vi "Updater Install DIAdem 2011.vi"(8 "error in (no error)":errorcluster, 11 "Spartan Install Path":path) -> (0 "error out":errorcluster)   [LabVIEW 2011]
uses:
  <vilib>/registry/registry.llb/Read Registry Value Simple STR.vi
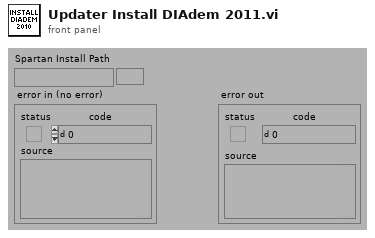
[diagram p1: front panel]
types:
  T1 = typedef "Registry refnum.ctl" = refnum<k1>
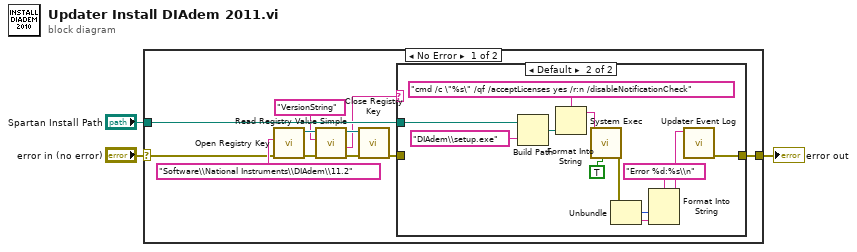
[diagram p0: block diagram]
diagram:
  n1 = case shown="No Error" "error in (no error)" {
    selector: "error in (no error)" -> [w4 w28]
    tunnel: [w14 w28] -> w3
    tunnel: "Spartan Install Path" -> [w13 _]
    frame No Error {
      n2 = call <vilib>:"Open Registry Key.vi"("error in (no error)"=w4, "subkey"="Software\\National Instruments\\DIAdem\\11.2") -> ("error out"=w10:errorcluster, "refnum out"=w9:T1)  [unwired: 8 in]
      n3 = call-poly <vilib>:"Read Registry Value Simple.vi"("error in (no error)"=w10, "value"="VersionString", "refnum"=w9) -> ("error out"=w6:errorcluster, "String/Binary data"=w5:string, "refnum out"=w7:T1)  [unwired: 3 in, 1 out]
      n4 = call <vilib>:"Close Registry Key.vi"("error in (no error)"=w6, "refnum"=w7) -> ("error out"=w12:errorcluster)  [unwired: 5 in]
      n5 = case shown="Default" w5 {
        tunnel: w12 -> [w15 _]
        tunnel: [w15 w16] -> w14
        tunnel: w13 -> [_ w27]
        frame "2010" {
        }
        frame Default {
          n6 = Build Path(base path=w27, name or relative path="DIAdem\\setup.exe") -> (appended path=w24:path)
          n7 = Format Into String(format string="cmd /c \"%s\" /qf /acceptLicenses yes /r:n /disableNotificationCheck", w24) -> (resulting string=w22:string)  [unwired: 2 in, 1 out]
          n8 = call <vilib>:"System Exec.vi"("run minimized? (F)"=TRUE, "command line"=w22) -> ("error out"=w17:errorcluster)  [unwired: 6 in, 3 out]
          n9 = Unbundle(w17) -> ("code"=w19:i32, "source"=w20:string)  [unwired: 1 out]
          n10 = Format Into String(format string="Error %d:%s\\n" ("pattern"), w19, w20) -> (resulting string=w21:string)  [unwired: 2 in, 1 out]
          n11 = call "Updater Event Log.vi"("Log Entry"=w21) -> ("error out"=w16:errorcluster)  [unwired: 1 in, 9 out]
        }
      }
    }
    frame Error {
    }
  }
  "error out" <- w3
